vi "Fetch Waveform (1D I16 (unscaled)).vi"(8 "error in (no error)":errorcluster, 9 "Maximum Time (10000ms)":u32=10000, 10 "Channel (0: Channel 1)":u16(ring) items=["Channel 1", "Channel 2", "Channel 3", "Channel 4", "Math", "Reference 1", "Reference 2", "Reference 3", "Reference 4"], 11 "VISA resource name":refnum<visa-resource-name>) -> (0 "error out":errorcluster, 1 "I16":i8[](array[numeric]), 3 "VISA resource name out":refnum<visa-resource-name>, 5 "dt":dbl, 7 "t0":dbl)   [LabVIEW 2017, in "Scope.lvlib" / "Tektronix DPO MSO 2000 4000 Series.lvlib"]
doc: "Returns the raw data that an oscilloscope acquires for a channel you specify. An acquisition that you initiate before calling this VI generates the waveform. The waveform data you fetch from the oscilloscope is an interger value, expressed in waveform data point level. If data width is of one byte, the data range is 0 to 255. If data width is of two bytes, the data range is 0 to 65535. You choose to use this VI when you want a relative fast fetching speed as well as output data expressed in waveform data point level. If you want output waveform data expressed in unit of volts, you could use this VI and manually scale the output data, or you could choose to use the <B>Fetch Waveform(Waveform Data Type)</B> VI.\n\nYou first enable channels with the Configure Channel VI. Then you use the Initiate VI to start an acquisition on the enabled channels. An oscilloscope concurrently acquires waveforms for these channels. You must call the Fetch Waveform VI separately to obtain waveforms for each enabled channel.\nHowever, you also can call the Read Waveform VI instead of using the above low-level VIs.\n\n<B>Note</B>: Use the Fetch Waveform VI only with other low-level VIs, such as the Initiate VI, the Abort VI, and the Fetch Waveform Measurement VI. High-level VIs, such as the Read Waveform VI, automatically incorporate the functions of the Initiate VI and the Fetch Waveform VI. The Fetch Waveform VI does not check the status of an instrument."
uses:
  Tektronix DPO MSO 2000 4000 Series.lvlib
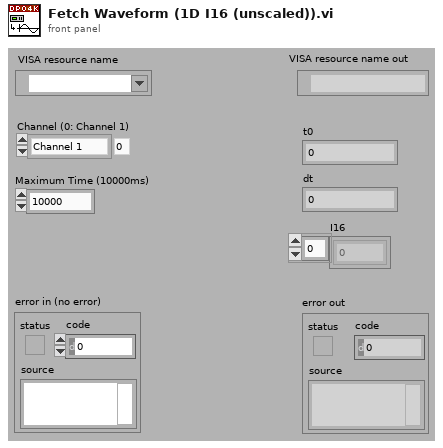
[diagram p1: front panel]
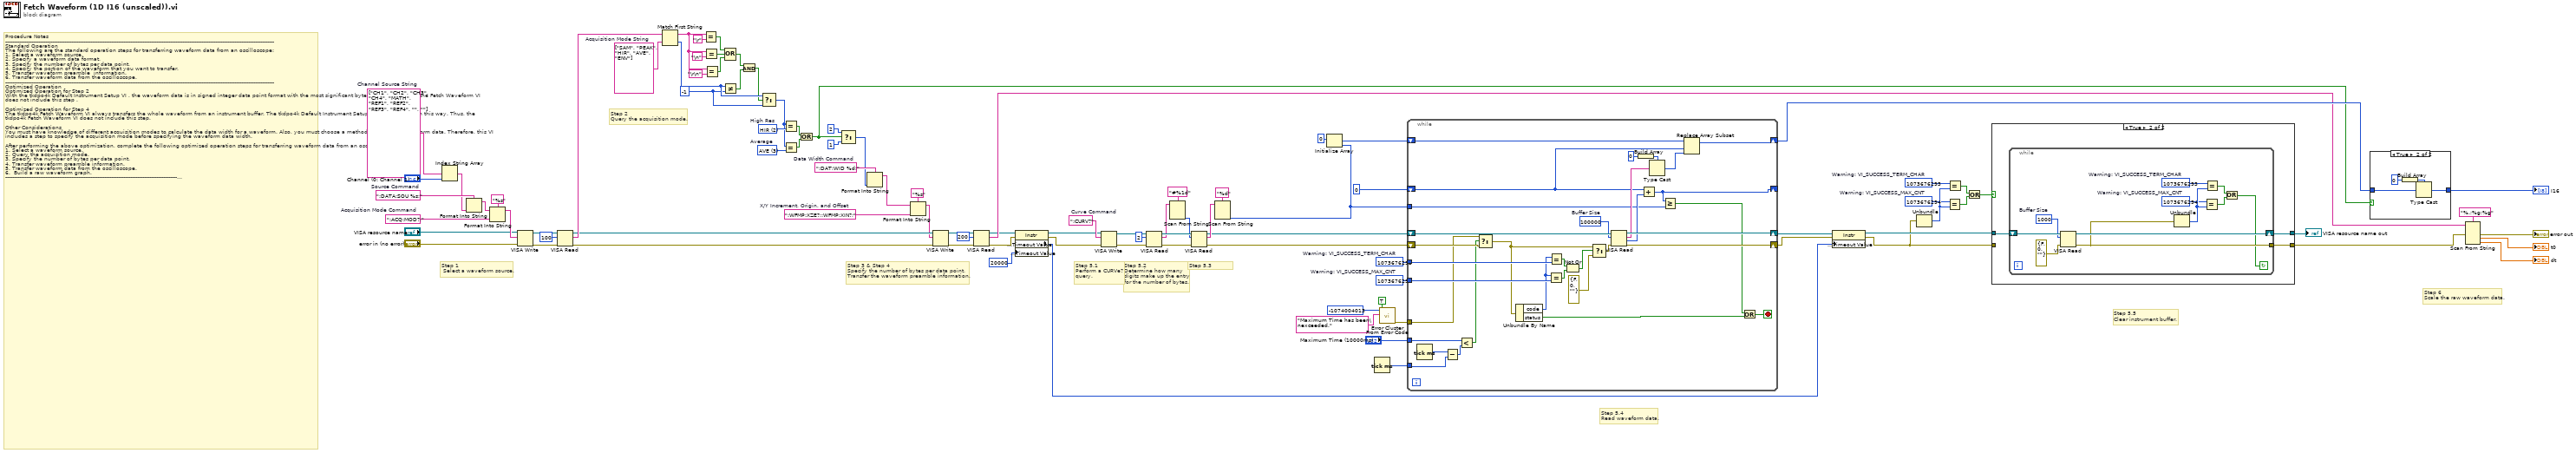
[diagram p0: block diagram]
diagram:
  w30 = ":WFMP:XZE?;:WFMP:XIN?;"  # X/Y Increment, Origin, and Offset
  w40 = 1073676294  # Warning: VI_SUCCESS_MAX_CNT
  w41 = 1073676293  # Warning: VI_SUCCESS_TERM_CHAR
  w44 = 1073676294  # Warning: VI_SUCCESS_MAX_CNT
  w43 = 1073676293  # Warning: VI_SUCCESS_TERM_CHAR
  w53 = -1 ("y")
  w79 = ":CURV?"  # Curve Command
  w81 = ":DAT:WID %d;"  # Data Width Command
  w86 = u16 3 items=["SAM", "PEAK", "HIR", "AVE", "ENV"]  # Average
  w87 = u16 2 items=["SAM", "PEAK", "HIR", "AVE", "ENV"]  # High Res
  w65 = string[] ["SAM", "PEAK", "HIR", "AVE", "ENV"]  # Acquisition Mode String
  w80 = ":ACQ:MOD?;"  # Acquisition Mode Command
  w96 = string[] ["CH1", "CH2", "CH3", "CH4", "MATH", "REF1", "REF2", "REF3", "REF4", "", ""]  # Channel Source String
  w95 = ":DATA:SOU %s;"  # Source Command
  # "Step 6    \nScale the raw waveform data."
  # "Step 5.5    \nClear instrument buffer."
  # "Step 5.4   \nRead waveform data."
  # "Step 5.3"
  # "Step 5.2      \nDetermine how many \ndigits make up the entry\nfor the number of bytes."
  # "Step 5.1      \nPerform a CURVe?\nquery."
  # "Step 3 & Step 4         \nSpecify the number of bytes per data point.\nTransfer the waveform preamble information."
  # "Step 2\nQuery the acquisition mode."
  # "Step 1        \n Select a waveform source."
  # "Procedure Notes\n-----------------------------------------------------------------------------------------------------------------------------------------------------------\nStandard Operation\nThe following are the standard operation steps for transferring waveform data from an oscilloscope:\n1. Select a waveform source.\n2. Specify a waveform data format.\n3. Specify the number of bytes per data point.\n4. Specify the portion of the waveform that you want to transfer.\n5. Transfer waveform preamble  information.\n6. Transfer waveform data from the oscilloscope.\n-----------------------------------------------------------------------------------------------------------------------------------------------------------\nOptimized Operation\nOptimized Operation for Step 2\nWith the tkdpo4k Default Instrument Setup VI , the waveform data is in signed integer data point format with the most significant byte transfer first. Thus, the Fetch Waveform VI does not include this step . \n\nOptimized Operation for Step 4 \nThe tkdpo4k Fetch Waveform VI always transfers the whole waveform from an instrument buffer. The tkdpo4k Default Instrument Setup VI  also operates in this way. Thus, the tkdpo4k Fetch Waveform VI does not include this step. \n\nOther Considerations\nYou must have knowledge of different acquisition modes to calculate the data width for a waveform. Also, you must choose a method to scale raw waveform data. Therefore, this VI includes a step to specify the acquisition mode before specifying the waveform data width.\n\nAfter performing the above optimization, complete the following optimized operation steps for transferring waveform data from an oscilloscope:\n1. Select a waveform source.\n2. Query the acquisition mode.\n3. Specify the number of bytes per data point.\n4. Transfer waveform preamble information.\n5. Transfer waveform data from the oscilloscope.\n6.  Build a raw waveform graph.\n-----------------------------------------------------------------------------------------------------------------------------------------------------------\nDetailed Steps\nThe following steps detail the behavior of this VI:\n1. Select a waveform source. \n2. Query and determine the acquisition mode. A correct determination is critical to steps 3 and 6.\n    -----------------------------------------------\n    Acquisition Mode |  Data Width  \n    -----------------------------------------------\n    Normal                       | 1                    \n    -----------------------------------------------\n    Peak Detect               | 1                   \n    -----------------------------------------------\n    Hi Res                        | 2                    \n    -----------------------------------------------\n    Envelope                   | 1                   \n    -----------------------------------------------\n    Average                    | 2                     \n    -----------------------------------------------\n3. Specify the number of bytes per data point. For the Hi Res or Average acquisition modes, set the data width to 2. For all other acquisition modes, set the data width to 1.\n4. Transfer the waveform preamble information. Necessary preamble information includes XZero, XIncrement. This VI uses XZero and XIncrement to configure the x-axis of output waveforms.\n5. Transfer waveform data from the oscilloscope.\n    5.1 Perform a CURVe? query.\n    5.2 Determine how many digits make up the entry for the number of bytes.\n    5.3 Read the data size.\n    5.4 Call the VISA Read VI repeatedly with a buffer size of 10000 until you obtain as much data as the data size specifies. Use      an 8-bit array to store the raw waveform data you obtain. \n    5.5 Continue reading the data remaining in the instrument buffer until the buffer is empty.\n6. Build a raw waveform graph."
  n1 = Index String Array(1:"Channel (0: Channel 1)", 2:w96) -> (0:w94:string)  [unwired: 1 in]
  n2 = Format Into String(format string=w95, w94) -> (resulting string=w93:string)  [unwired: 2 in, 1 out]
  n3 = Format Into String(format string="%s", initial string=w93, w80) -> (resulting string=w91:string)  [unwired: 1 in, 1 out]
  n4 = VISA Write(VISA resource name="VISA resource name", write buffer=w91, error in (no error)="error in (no error)") -> (VISA resource name out=w90:refnum<visa-resource-name>, error out=w89:errorcluster)  [unwired: 1 out]
  n5 = VISA Read(VISA resource name=w90, byte count=u32 100, error in (no error)=w89) -> (VISA resource name out=w34:refnum<visa-resource-name>, read buffer=w64:string, error out=w33:errorcluster)  [unwired: 1 out]
  n6 = Match First String(2:w65, 3:w64) -> (0:w54:i32, 1:w60:string)
  n7 = Equal?(x=w60, y="\r") -> (x = y?=w59:bool)
  n8 = Equal?(x=w60, y="\n") -> (x = y?=w58:bool)
  n9 = Equal?(x=w60, y="\r\n") -> (x = y?=w57:bool)
  n10 = Not Equal?(x=w54, y=w53) -> (x != y?=w55:bool)
  n11 = Compound Arithmetic op=OR(w59, w58, w57) -> (w56:bool)
  n12 = And(x=w56, y=w55) -> (x .and. y?=w52:bool)
  n13 = Select(t=w54, s=w52, f=w53) -> (s? t:f=w32:i32)
  n14 = Equal?(x=w32, y=w87) -> (x = y?=w85:bool)
  n15 = Equal?(x=w32, y=w86) -> (x = y?=w84:bool)
  n16 = Or(x=w85, y=w84) -> (x .or. y?=w14:bool)
  n17 = Select(t=2 ("f"), s=w14, f=1) -> (s? t:f=w68:i32)
  n18 = Format Into String(format string=w81, w68) -> (resulting string=w29:string)  [unwired: 2 in, 1 out]
  n19 = Format Into String(format string="%s", initial string=w29, w30) -> (resulting string=w28:string)  [unwired: 1 in, 1 out]
  n20 = VISA Write(VISA resource name=w34, write buffer=w28, error in (no error)=w33) -> (VISA resource name out=w27:refnum<visa-resource-name>, error out=w26:errorcluster)  [unwired: 1 out]
  n21 = VISA Read(VISA resource name=w27, byte count=u32 200, error in (no error)=w26) -> (VISA resource name out=w6:refnum<visa-resource-name>, read buffer=w25:string, error out=w4:errorcluster)  [unwired: 1 out]
  n22 = property class="Instr"(reference=w6, error in=w4, "General Settings:Timeout Value"=u32 20000) -> (reference out=w5:refnum<visa-resource-name>, error out=w3:errorcluster, "General Settings:Timeout Value"=w18:u32)
  n23 = VISA Write(VISA resource name=w5, write buffer=w79, error in (no error)=w3) -> (VISA resource name out=w77:refnum<visa-resource-name>, error out=w78:errorcluster)  [unwired: 1 out]
  n24 = VISA Read(VISA resource name=w77, byte count=u32 2, error in (no error)=w78) -> (VISA resource name out=w74:refnum<visa-resource-name>, read buffer=w72:string, error out=w73:errorcluster)  [unwired: 1 out]
  n25 = Scan From String(format string="#%1d", input string=w72) -> (output 1=w71:i32)  [unwired: 3 in, 3 out]
  n26 = VISA Read(VISA resource name=w74, byte count=w71, error in (no error)=w73) -> (VISA resource name out=w2:refnum<visa-resource-name>, read buffer=w69:string, error out=w1:errorcluster)  [unwired: 1 out]
  n27 = Scan From String(format string="%d", input string=w69) -> (output 1=w51:i32)  [unwired: 3 in, 3 out]
  n28 = Initialize Array(i8 0 ("element"), w51) -> (w49:i8[])
  n29 = Tick Count (ms)() -> (millisecond timer value=w9:u32)
  n30 = call <vilib>:"Error Cluster From Error Code.vi"("show call chain? (False)"=TRUE, "error message (\"\")"="Maximum Time has been\nexceeded." ("error message (\"\")"), "error code (0)"=-1074004013) -> ("error out"=w7:errorcluster)  [unwired: 6 in]
  n31 = while {
    shift-right: [w127] -> w22
    shift-left: w2 -> [w129]
    shift-right: [w126] -> w21
    shift-left: w1 -> [w99]
    shift-right: [w122] -> w67
    shift-left: w49 -> [w123]
    tunnel: w51 -> [w119]
    shift-right: [w116] -> _
    shift-left: 0 -> [w117]
    tunnel: w41 -> [w110]
    tunnel: w40 -> [w109]
    tunnel: w9 -> [w102]
    tunnel: "Maximum Time (10000ms)" -> [w101]
    tunnel: w7 -> [w97]
    stop <- w115 stop-if-true
    w128 = 100000  # Buffer Size
    n32 = Tick Count (ms)() -> (millisecond timer value=w103:u32)
    n33 = Subtract(x=w103, y=w102) -> (x-y=w104:u32)
    n34 = Less?(x=w101, y=w104) -> (x < y?=w98:bool)
    n35 = Select(t=w97, s=w98, f=w99) -> (s? t:f=w100:errorcluster)
    n36 = Unbundle By Name(w100) -> ("code"=w108:i32, "status"=w112:bool)
    n37 = Equal?(x=w108, y=w109) -> (x = y?=w106:bool)
    n38 = Equal?(x=w108, y=w110) -> (x = y?=w107:bool)
    n39 = Not Or(1:w106, 2:w107) -> (0:w105:bool)
    n40 = Select(t=w100, s=w105, f=errorcluster {"status"=FALSE, "code"=0, "source"=""} ("error in (no error)")) -> (s? t:f=w111:errorcluster)
    n41 = VISA Read(VISA resource name=w129, byte count=w128, error in (no error)=w111) -> (VISA resource name out=w127:refnum<visa-resource-name>, read buffer=w121:string, return count=w120:u32, error out=w126:errorcluster)
    n42 = Build Array(i8 0) -> (w125:i8[])
    n43 = Add(x=w117, y=w120) -> (x+y=w116:u32)
    n44 = Type Cast(type=w125, x=w121) -> (*(type *) &x=w118:i8[])
    n45 = Greater Or Equal?(x=w116, y=w119) -> (x >= y?=w114:bool)
    n46 = Replace Array Subset(array=w123, new element=w118, index=w117) -> (w122:i8[])
    n47 = Or(x=w114, y=w112) -> (x .or. y?=w115:bool)
  }
  n48 = property class="Instr"(reference=w22, error in=w21, "General Settings:Timeout Value"=w18) -> (reference out=w20:refnum<visa-resource-name>, error out=w19:errorcluster)
  n49 = Unbundle(w19) -> ("code"=w45:i32)  [unwired: 2 out]
  n50 = Equal?(x=w44, y=w45) -> (x = y?=w47:bool)
  n51 = Equal?(x=w43, y=w45) -> (x = y?=w48:bool)
  n52 = Or(x=w48, y=w47) -> (x .or. y?=w46:bool)
  n53 = case shown="True" w46 {
    tunnel: w20 -> [w131 w134]
    tunnel: w19 -> [w130 _]
    tunnel: [w131 w133] -> w36
    tunnel: [w130 w132] -> w66
    frame False {
    }
    frame True {
      n54 = while {
        shift-right: [w144] -> w133
        shift-left: w134 -> [w145]
        tunnel: [w137] -> w132
        stop <- w136 continue-if-true
        w139 = 1073676294  # Warning: VI_SUCCESS_MAX_CNT
        w138 = 1073676293  # Warning: VI_SUCCESS_TERM_CHAR
        w143 = u32 1000  # Buffer Size
        n55 = VISA Read(VISA resource name=w145, byte count=w143, error in (no error)=errorcluster {"status"=FALSE, "code"=0, "source"=""}) -> (VISA resource name out=w144:refnum<visa-resource-name>, error out=w137:errorcluster)  [unwired: 2 out]
        n56 = Unbundle(w137) -> ("code"=w140:i32)  [unwired: 2 out]
        n57 = Equal?(x=w139, y=w140) -> (x = y?=w141:bool)
        n58 = Equal?(x=w138, y=w140) -> (x = y?=w142:bool)
        n59 = Or(x=w142, y=w141) -> (x .or. y?=w136:bool)
      }
    }
  }
  "VISA resource name out" <- w36
  n60 = case shown="True" w14 {
    tunnel: w67 -> [w146 w150]
    tunnel: [w146 w147] -> w13
    frame False {
    }
    frame True {
      n61 = Build Array(i16 0 ("element")) -> (w148:i16[])
      n62 = Type Cast(type=w148, x=w150) -> (*(type *) &x=w147:i16[])
    }
  }
  "I16" <- w13
  n63 = Scan From String(format string="%.;%g;%g", input string=w25, error in=w66) -> (error out=→"error out":errorcluster, output 1=→"t0":dbl, output 2=→"dt":dbl)  [unwired: 3 in, 2 out]
